vi "Insts_init.vi"(2 "Initialize sweep instruments ??":u64[](array[numeric]), 3 "sweep_list":string[](array[string])=["0:0"], 4 "Initialize readout instruments??":u64[](array[numeric]), 5 "Inst_array":T2(array[cluster])) -> (0 "Sweep inst parameters":T1(array[cluster]), 1 "Readout inst parameters":T1(array[cluster]))   [LabVIEW 2013]
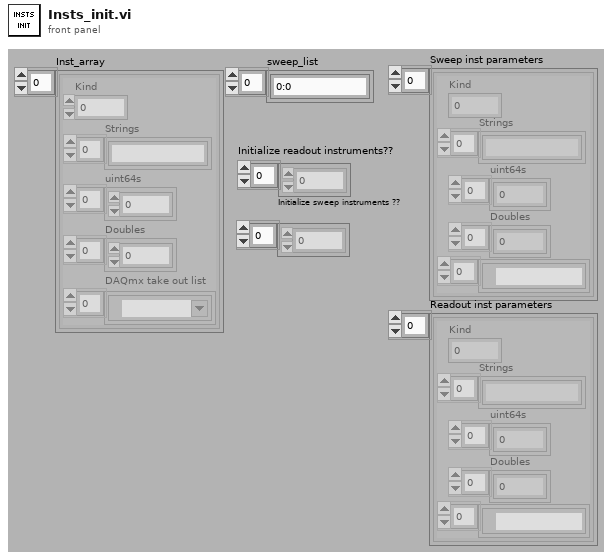
[diagram p1: front panel]
types:
  T1 = cluster{"Kind":u16, "Strings":string[], "uint64s":u64[], "Doubles":dbl[], refnum<k21>[]}[]
  T2 = cluster{"Kind":u16, "Strings":string[], "uint64s":u64[], "Doubles":dbl[], "DAQmx take out list":refnum<k21>[]}[]
  T3 = cluster{"Kind":u16, "Strings":string[], "uint64s":u64[], "Doubles":dbl[], refnum<k21>[]}
  T4 = cluster{"Kind":u16, "Strings":string[], "uint64s":u64[], "Doubles":dbl[], "DAQmx take out list":refnum<k21>[]}
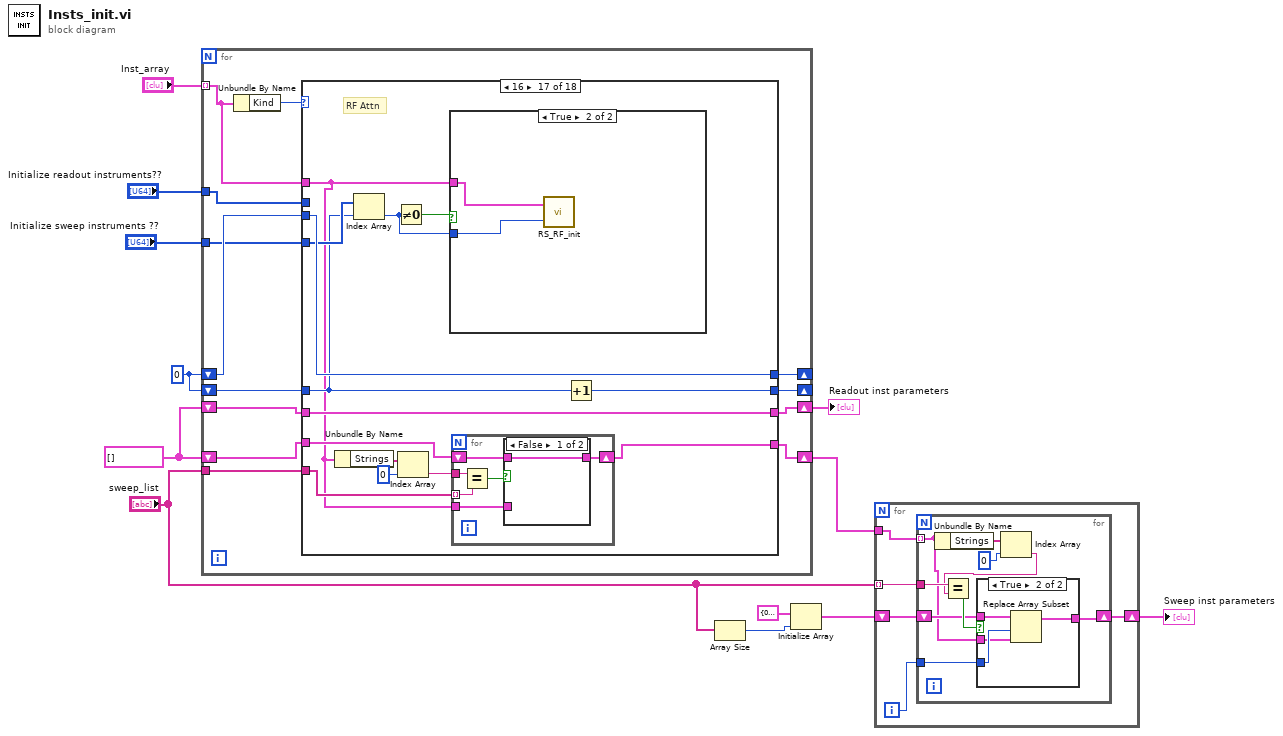
[diagram p0: block diagram]
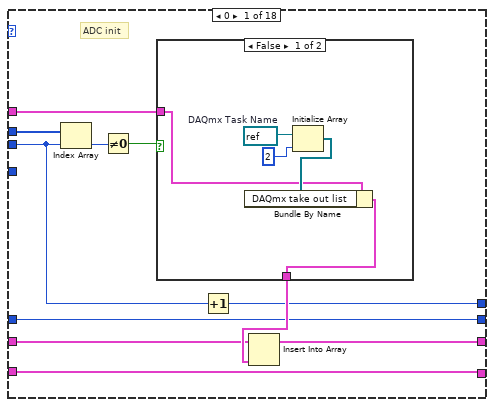
[diagram p3: hidden frame]
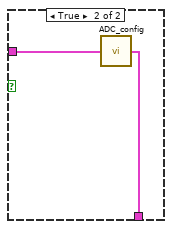
[diagram p4: hidden frame]
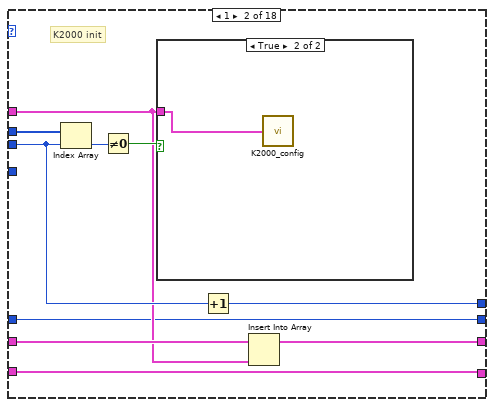
[diagram p5: hidden frame]
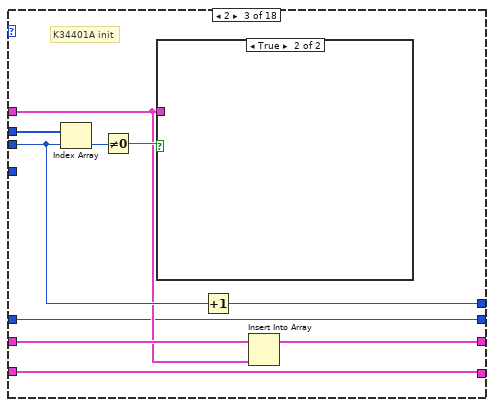
[diagram p7: hidden frame]
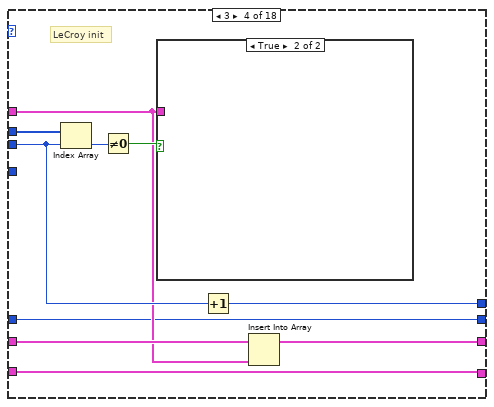
[diagram p9: hidden frame]
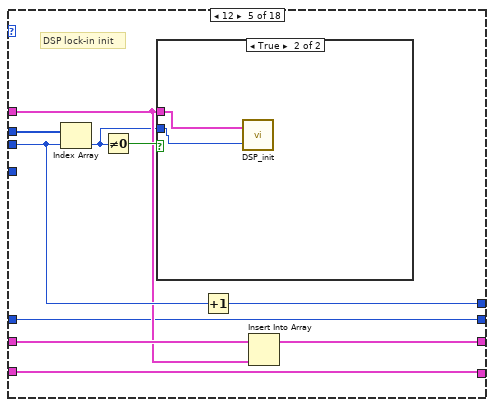
[diagram p11: hidden frame]
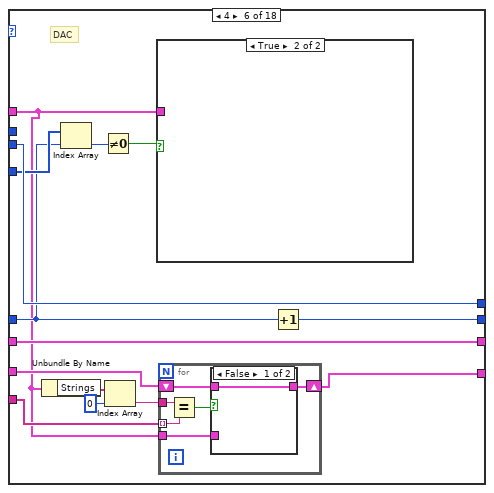
[diagram p13: hidden frame]
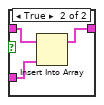
[diagram p14: hidden frame]
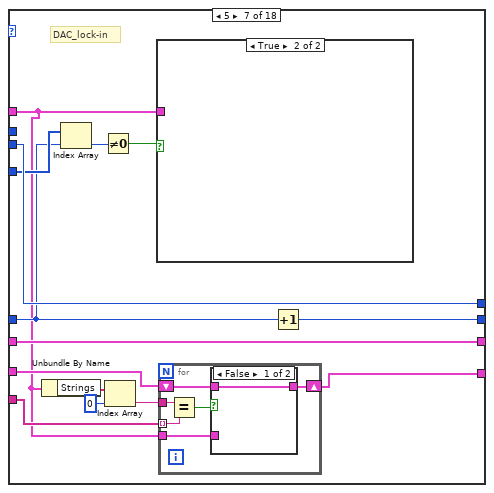
[diagram p16: hidden frame]
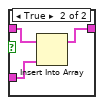
[diagram p17: hidden frame]
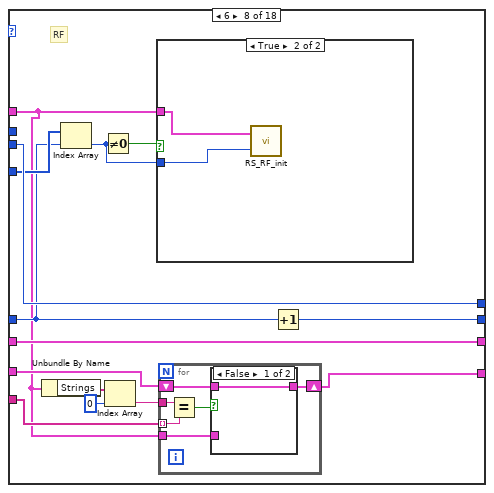
[diagram p19: hidden frame]
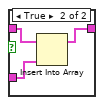
[diagram p20: hidden frame]
diagram:
  w9 = 0
  w8 = T1 [] ("Readout parameters")
  n1 = for {
    tunnel: "Inst_array" -> [w22] mode=indexing
    tunnel: "Initialize sweep instruments ??" -> [w19]
    tunnel: "Initialize readout instruments??" -> [w23]
    shift-right: [w13] -> w7
    shift-left: w8 -> [w16]
    shift-right: [w14] -> w2
    shift-left: w8 -> [w15]
    shift-right: [w21] -> _
    shift-left: w9 -> [w24]
    shift-right: [w18] -> _
    shift-left: w9 -> [w20]
    tunnel: "sweep_list" -> [w17]
    n2 = Unbundle By Name(w22) -> ("Kind"=w25:u16)
    n3 = case shown="16" w25 {
      tunnel: w24 -> [w31 w50 w61 w71 w82 w98 w122 w147 w173 w199 w223 w247 w271 w295 w319 w343 w369 w386]
      tunnel: w23 -> [w36 w53 w64 w74 w84 _ _ _ _ _ _ _ _ _ _ _ _ _]
      tunnel: w22 -> [w33 w46 w57 w67 w78 w87 w111 w136 w162 w188 w212 w236 w260 w284 w308 w332 w358 _]
      tunnel: [w30 w49 w60 w70 w81 w98 w122 w147 w173 w199 w223 w247 w271 w295 w319 w343 w369 w386] -> w21
      tunnel: w16 -> [w29 w48 w59 w69 w80 w95 w119 w144 w170 w196 w220 w244 w268 w292 w316 w340 w366 w385]
      tunnel: [w28 w47 w58 w68 w79 w95 w119 w144 w170 w196 w220 w244 w268 w292 w316 w340 w366 w385] -> w13
      tunnel: w20 -> [w27 w45 w56 w66 w77 w94 w118 w143 w169 w195 w219 w243 w267 w291 w315 w339 w365 w384]
      tunnel: w19 -> [_ _ _ _ _ w97 w121 w146 w172 w198 w222 w246 w270 w294 w318 w342 w368 _]
      tunnel: [w27 w45 w56 w66 w77 w96 w120 w145 w171 w197 w221 w245 w269 w293 w317 w341 w367 w384] -> w18
      tunnel: w15 -> [w26 w44 w55 w65 w76 w89 w113 w138 w164 w190 w214 w238 w262 w286 w310 w334 w360 w383]
      tunnel: [w26 w44 w55 w65 w76 w88 w112 w137 w163 w189 w213 w237 w261 w285 w309 w333 w359 w383] -> w14
      tunnel: w17 -> [_ _ _ _ _ w90 w114 w139 w165 w191 w215 w239 w263 w287 w311 w335 w361 _]
      frame 0 {
        # "ADC init"
        n4 = Index Array(array=w36, index=w31) -> (element=w35:u64)
        n5 = Not Equal To 0?(x=w35) -> (x != 0?=w34:bool)
        n6 = case shown="False" w34 {
          tunnel: w33 -> [w38 w43]
          tunnel: [w37 w42] -> w32
          frame False {
            w41 = refnum<k21> refnum  # DAQmx Task Name
            n7 = Initialize Array(w41, 2) -> (w39:refnum<k21>[])
            n8 = Bundle By Name(cluster=w38, "DAQmx take out list"=w39) -> (w37:T4)
          }
          frame True {
            n9 = call "ADC_config.vi"("Inst_parameter"=w43) -> ("Inst_parameter out"=w42:T4)
          }
        }
        n10 = Increment(x=w31) -> (x+1=w30:i32)
        n11 = Insert Into Array(array=w29, new element=w32) -> (w28:T1)  [unwired: 1 in]
      }
      frame 1 {
        # "K2000 init"
        n12 = Index Array(array=w53, index=w50) -> (element=w52:u64)
        n13 = Not Equal To 0?(x=w52) -> (x != 0?=w51:bool)
        n14 = case shown="True" w51 {
          tunnel: w46 -> [_ w54]
          frame False {
          }
          frame True {
            n15 = call "K2000_config.vi"("Readout_inst_parameters"=w54) -> ()  [unwired: 1 out]
          }
        }
        n16 = Increment(x=w50) -> (x+1=w49:i32)
        n17 = Insert Into Array(array=w48, new element=w46) -> (w47:T1)  [unwired: 1 in]
      }
      frame 2 {
        # "K34401A init"
        n18 = Index Array(array=w64, index=w61) -> (element=w63:u64)
        n19 = Not Equal To 0?(x=w63) -> (x != 0?=w62:bool)
        n20 = case shown="True" w62 {
          tunnel: w57 -> [_ _]
          frame False {
          }
          frame True {
          }
        }
        n21 = Increment(x=w61) -> (x+1=w60:i32)
        n22 = Insert Into Array(array=w59, new element=w57) -> (w58:T1)  [unwired: 1 in]
      }
      frame 3 {
        # "LeCroy init"
        n23 = Index Array(array=w74, index=w71) -> (element=w73:u64)
        n24 = Not Equal To 0?(x=w73) -> (x != 0?=w72:bool)
        n25 = case shown="True" w72 {
          tunnel: w67 -> [_ _]
          frame False {
          }
          frame True {
          }
        }
        n26 = Increment(x=w71) -> (x+1=w70:i32)
        n27 = Insert Into Array(array=w69, new element=w67) -> (w68:T1)  [unwired: 1 in]
      }
      frame 12 {
        # "DSP lock-in init"
        n28 = Index Array(array=w84, index=w82) -> (element=w75:u64)
        n29 = Not Equal To 0?(x=w75) -> (x != 0?=w83:bool)
        n30 = case shown="True" w83 {
          tunnel: w78 -> [_ w86]
          tunnel: w75 -> [_ w85]
          frame False {
          }
          frame True {
            n31 = call "DSP_init.vi"("Initialize Instrument"=w85, "Inst_param"=w86) -> ()  [unwired: 1 in]
          }
        }
        n32 = Increment(x=w82) -> (x+1=w81:i32)
        n33 = Insert Into Array(array=w80, new element=w78) -> (w79:T1)  [unwired: 1 in]
      }
      frame 4 {
        # "DAC"
        n34 = Unbundle By Name(w87) -> ("Strings"=w93:string[])
        n35 = Index Array(array=w97, index=w94) -> (element=w100:u64)
        n36 = Not Equal To 0?(x=w100) -> (x != 0?=w99:bool)
        n37 = Index Array(array=w93, index=0) -> (element=w91:string)
        n38 = case shown="True" w99 {
          tunnel: w87 -> [_ _]
          frame False {
          }
          frame True {
          }
        }
        n39 = for {
          tunnel: w91 -> [w106]
          tunnel: w90 -> [w105] mode=indexing
          shift-right: [w101] -> w88
          shift-left: w89 -> [w102]
          tunnel: w87 -> [w103]
          n40 = Equal?(x=w106, y=w105) -> (x = y?=w104:bool)
          n41 = case shown="False" w104 {
            tunnel: w103 -> [_ w110]
            tunnel: w102 -> [w107 w109]
            tunnel: [w107 w108] -> w101
            frame False {
            }
            frame True {
              n42 = Insert Into Array(array=w109, new element=w110) -> (w108:T1)  [unwired: 1 in]
            }
          }
        }
        n43 = Increment(x=w94) -> (x+1=w96:i32)
      }
      frame 5 {
        # "DAC_lock-in"
        n44 = Unbundle By Name(w111) -> ("Strings"=w117:string[])
        n45 = Index Array(array=w121, index=w118) -> (element=w124:u64)
        n46 = Not Equal To 0?(x=w124) -> (x != 0?=w123:bool)
        n47 = Index Array(array=w117, index=0) -> (element=w115:string)
        n48 = case shown="True" w123 {
          tunnel: w111 -> [_ _]
          frame False {
          }
          frame True {
          }
        }
        n49 = for {
          tunnel: w115 -> [w130]
          tunnel: w114 -> [w129] mode=indexing
          shift-right: [w125] -> w112
          shift-left: w113 -> [w126]
          tunnel: w111 -> [w127]
          n50 = Equal?(x=w130, y=w129) -> (x = y?=w128:bool)
          n51 = case shown="False" w128 {
            tunnel: w127 -> [_ w134]
            tunnel: w126 -> [w131 w133]
            tunnel: [w131 w132] -> w125
            frame False {
            }
            frame True {
              n52 = Insert Into Array(array=w133, new element=w134) -> (w132:T1)  [unwired: 1 in]
            }
          }
        }
        n53 = Increment(x=w118) -> (x+1=w120:i32)
      }
      frame 6 {
        # "RF"
        n54 = Unbundle By Name(w136) -> ("Strings"=w142:string[])
        n55 = Index Array(array=w146, index=w143) -> (element=w135:u64)
        n56 = Not Equal To 0?(x=w135) -> (x != 0?=w148:bool)
        n57 = Index Array(array=w142, index=0) -> (element=w140:string)
        n58 = case shown="True" w148 {
          tunnel: w136 -> [_ w160]
          tunnel: w135 -> [_ w159]
          frame False {
          }
          frame True {
            n59 = call "RS_RF_init.vi"("Initialize Instrument"=w159, "Inst_param"=w160) -> ()  [unwired: 1 in]
          }
        }
        n60 = for {
          tunnel: w140 -> [w154]
          tunnel: w139 -> [w153] mode=indexing
          shift-right: [w149] -> w137
          shift-left: w138 -> [w150]
          tunnel: w136 -> [w151]
          n61 = Equal?(x=w154, y=w153) -> (x = y?=w152:bool)
          n62 = case shown="False" w152 {
            tunnel: w151 -> [_ w158]
            tunnel: w150 -> [w155 w157]
            tunnel: [w155 w156] -> w149
            frame False {
            }
            frame True {
              n63 = Insert Into Array(array=w157, new element=w158) -> (w156:T1)  [unwired: 1 in]
            }
          }
        }
        n64 = Increment(x=w143) -> (x+1=w145:i32)
      }
      frame 7 {
        # "AWG"
        n65 = Unbundle By Name(w162) -> ("Strings"=w168:string[])
        n66 = Index Array(array=w172, index=w169) -> (element=w161:u64)
        n67 = Not Equal To 0?(x=w161) -> (x != 0?=w174:bool)
        n68 = Index Array(array=w168, index=0) -> (element=w166:string)
        n69 = case shown="True" w174 {
          tunnel: w162 -> [_ w186]
          tunnel: w161 -> [_ w185]
          frame False {
          }
          frame True {
            n70 = call "AWG_init.vi"("Initialize?"=w185, "Inst_param"=w186) -> ()  [unwired: 1 out]
          }
        }
        n71 = for {
          tunnel: w166 -> [w180]
          tunnel: w165 -> [w179] mode=indexing
          shift-right: [w175] -> w163
          shift-left: w164 -> [w176]
          tunnel: w162 -> [w177]
          n72 = Equal?(x=w180, y=w179) -> (x = y?=w178:bool)
          n73 = case shown="False" w178 {
            tunnel: w177 -> [_ w184]
            tunnel: w176 -> [w181 w183]
            tunnel: [w181 w182] -> w175
            frame False {
            }
            frame True {
              n74 = Insert Into Array(array=w183, new element=w184) -> (w182:T1)  [unwired: 1 in]
            }
          }
        }
        n75 = Increment(x=w169) -> (x+1=w171:i32)
      }
      frame 8 {
        # "B-field"
        n76 = Unbundle By Name(w188) -> ("Strings"=w194:string[])
        n77 = Index Array(array=w198, index=w195) -> (element=w187:u64)
        n78 = Not Equal To 0?(x=w187) -> (x != 0?=w200:bool)
        n79 = Index Array(array=w194, index=0) -> (element=w192:string)
        n80 = case shown="True" w200 {
          tunnel: w188 -> [_ _]
          tunnel: w187 -> [_ _]
          frame False {
          }
          frame True {
          }
        }
        n81 = for {
          tunnel: w192 -> [w206]
          tunnel: w191 -> [w205] mode=indexing
          shift-right: [w201] -> w189
          shift-left: w190 -> [w202]
          tunnel: w188 -> [w203]
          n82 = Equal?(x=w206, y=w205) -> (x = y?=w204:bool)
          n83 = case shown="False" w204 {
            tunnel: w203 -> [_ w210]
            tunnel: w202 -> [w207 w209]
            tunnel: [w207 w208] -> w201
            frame False {
            }
            frame True {
              n84 = Insert Into Array(array=w209, new element=w210) -> (w208:T1)  [unwired: 1 in]
            }
          }
        }
        n85 = Increment(x=w195) -> (x+1=w197:i32)
      }
      frame 9 {
        # "Fast sequence"
        n86 = Unbundle By Name(w212) -> ("Strings"=w218:string[])
        n87 = Index Array(array=w222, index=w219) -> (element=w211:u64)
        n88 = Not Equal To 0?(x=w211) -> (x != 0?=w224:bool)
        n89 = Index Array(array=w218, index=0) -> (element=w216:string)
        n90 = case shown="True" w224 {
          tunnel: w212 -> [_ _]
          tunnel: w211 -> [_ _]
          frame False {
          }
          frame True {
          }
        }
        n91 = for {
          tunnel: w216 -> [w230]
          tunnel: w215 -> [w229] mode=indexing
          shift-right: [w225] -> w213
          shift-left: w214 -> [w226]
          tunnel: w212 -> [w227]
          n92 = Equal?(x=w230, y=w229) -> (x = y?=w228:bool)
          n93 = case shown="False" w228 {
            tunnel: w227 -> [_ w234]
            tunnel: w226 -> [w231 w233]
            tunnel: [w231 w232] -> w225
            frame False {
            }
            frame True {
              n94 = Insert Into Array(array=w233, new element=w234) -> (w232:T1)  [unwired: 1 in]
            }
          }
        }
        n95 = Increment(x=w219) -> (x+1=w221:i32)
      }
      frame 10 {
        # "Fast sequence slot"
        n96 = Unbundle By Name(w236) -> ("Strings"=w242:string[])
        n97 = Index Array(array=w246, index=w243) -> (element=w235:u64)
        n98 = Not Equal To 0?(x=w235) -> (x != 0?=w248:bool)
        n99 = Index Array(array=w242, index=0) -> (element=w240:string)
        n100 = case shown="True" w248 {
          tunnel: w236 -> [_ _]
          tunnel: w235 -> [_ _]
          frame False {
          }
          frame True {
          }
        }
        n101 = for {
          tunnel: w240 -> [w254]
          tunnel: w239 -> [w253] mode=indexing
          shift-right: [w249] -> w237
          shift-left: w238 -> [w250]
          tunnel: w236 -> [w251]
          n102 = Equal?(x=w254, y=w253) -> (x = y?=w252:bool)
          n103 = case shown="False" w252 {
            tunnel: w251 -> [_ w258]
            tunnel: w250 -> [w255 w257]
            tunnel: [w255 w256] -> w249
            frame False {
            }
            frame True {
              n104 = Insert Into Array(array=w257, new element=w258) -> (w256:T1)  [unwired: 1 in]
            }
          }
        }
        n105 = Increment(x=w243) -> (x+1=w245:i32)
      }
      frame 11 {
        # "Command line"
        n106 = Unbundle By Name(w260) -> ("Strings"=w266:string[])
        n107 = Index Array(array=w270, index=w267) -> (element=w259:u64)
        n108 = Not Equal To 0?(x=w259) -> (x != 0?=w272:bool)
        n109 = Index Array(array=w266, index=0) -> (element=w264:string)
        n110 = case shown="True" w272 {
          tunnel: w260 -> [_ _]
          tunnel: w259 -> [_ _]
          frame False {
          }
          frame True {
          }
        }
        n111 = for {
          tunnel: w264 -> [w278]
          tunnel: w263 -> [w277] mode=indexing
          shift-right: [w273] -> w261
          shift-left: w262 -> [w274]
          tunnel: w260 -> [w275]
          n112 = Equal?(x=w278, y=w277) -> (x = y?=w276:bool)
          n113 = case shown="False" w276 {
            tunnel: w275 -> [_ w282]
            tunnel: w274 -> [w279 w281]
            tunnel: [w279 w280] -> w273
            frame False {
            }
            frame True {
              n114 = Insert Into Array(array=w281, new element=w282) -> (w280:T1)  [unwired: 1 in]
            }
          }
        }
        n115 = Increment(x=w267) -> (x+1=w269:i32)
      }
      frame 13 {
        # "DSP lock-in sweep"
        n116 = Unbundle By Name(w284) -> ("Strings"=w290:string[])
        n117 = Index Array(array=w294, index=w291) -> (element=w283:u64)
        n118 = Not Equal To 0?(x=w283) -> (x != 0?=w296:bool)
        n119 = Index Array(array=w290, index=0) -> (element=w288:string)
        n120 = case shown="True" w296 {
          tunnel: w284 -> [_ _]
          tunnel: w283 -> [_ _]
          frame False {
          }
          frame True {
          }
        }
        n121 = for {
          tunnel: w288 -> [w302]
          tunnel: w287 -> [w301] mode=indexing
          shift-right: [w297] -> w285
          shift-left: w286 -> [w298]
          tunnel: w284 -> [w299]
          n122 = Equal?(x=w302, y=w301) -> (x = y?=w300:bool)
          n123 = case shown="False" w300 {
            tunnel: w299 -> [_ w306]
            tunnel: w298 -> [w303 w305]
            tunnel: [w303 w304] -> w297
            frame False {
            }
            frame True {
              n124 = Insert Into Array(array=w305, new element=w306) -> (w304:T1)  [unwired: 1 in]
            }
          }
        }
        n125 = Increment(x=w291) -> (x+1=w293:i32)
      }
      frame 14 {
        # "ms to wait"
        n126 = Unbundle By Name(w308) -> ("Strings"=w314:string[])
        n127 = Index Array(array=w318, index=w315) -> (element=w307:u64)
        n128 = Not Equal To 0?(x=w307) -> (x != 0?=w320:bool)
        n129 = Index Array(array=w314, index=0) -> (element=w312:string)
        n130 = case shown="True" w320 {
          tunnel: w308 -> [_ _]
          tunnel: w307 -> [_ _]
          frame False {
          }
          frame True {
          }
        }
        n131 = for {
          tunnel: w312 -> [w326]
          tunnel: w311 -> [w325] mode=indexing
          shift-right: [w321] -> w309
          shift-left: w310 -> [w322]
          tunnel: w308 -> [w323]
          n132 = Equal?(x=w326, y=w325) -> (x = y?=w324:bool)
          n133 = case shown="False" w324 {
            tunnel: w323 -> [_ w330]
            tunnel: w322 -> [w327 w329]
            tunnel: [w327 w328] -> w321
            frame False {
            }
            frame True {
              n134 = Insert Into Array(array=w329, new element=w330) -> (w328:T1)  [unwired: 1 in]
            }
          }
        }
        n135 = Increment(x=w315) -> (x+1=w317:i32)
      }
      frame 15 {
        # "ATM delay line"
        n136 = Unbundle By Name(w332) -> ("Strings"=w338:string[])
        n137 = Index Array(array=w342, index=w339) -> (element=w331:u64)
        n138 = Not Equal To 0?(x=w331) -> (x != 0?=w344:bool)
        n139 = Index Array(array=w338, index=0) -> (element=w336:string)
        n140 = case shown="True" w344 {
          tunnel: w332 -> [_ w356]
          tunnel: w331 -> [_ w355]
          frame False {
          }
          frame True {
            n141 = call "DelayLineInit.vi"("Inst bool"=w355, "Inst_param"=w356) -> ()  [unwired: 1 in]
          }
        }
        n142 = for {
          tunnel: w336 -> [w350]
          tunnel: w335 -> [w349] mode=indexing
          shift-right: [w345] -> w333
          shift-left: w334 -> [w346]
          tunnel: w332 -> [w347]
          n143 = Equal?(x=w350, y=w349) -> (x = y?=w348:bool)
          n144 = case shown="False" w348 {
            tunnel: w347 -> [_ w354]
            tunnel: w346 -> [w351 w353]
            tunnel: [w351 w352] -> w345
            frame False {
            }
            frame True {
              n145 = Insert Into Array(array=w353, new element=w354) -> (w352:T1)  [unwired: 1 in]
            }
          }
        }
        n146 = Increment(x=w339) -> (x+1=w341:i32)
      }
      frame 16 {
        # "RF Attn"
        n147 = Unbundle By Name(w358) -> ("Strings"=w364:string[])
        n148 = Index Array(array=w368, index=w365) -> (element=w357:u64)
        n149 = Not Equal To 0?(x=w357) -> (x != 0?=w370:bool)
        n150 = Index Array(array=w364, index=0) -> (element=w362:string)
        n151 = case shown="True" w370 {
          tunnel: w358 -> [_ w382]
          tunnel: w357 -> [_ w381]
          frame False {
          }
          frame True {
            n152 = call "RS_RF_init.vi"("Initialize Instrument"=w381, "Inst_param"=w382) -> ()  [unwired: 1 in]
          }
        }
        n153 = for {
          tunnel: w362 -> [w376]
          tunnel: w361 -> [w375] mode=indexing
          shift-right: [w371] -> w359
          shift-left: w360 -> [w372]
          tunnel: w358 -> [w373]
          n154 = Equal?(x=w376, y=w375) -> (x = y?=w374:bool)
          n155 = case shown="False" w374 {
            tunnel: w373 -> [_ w380]
            tunnel: w372 -> [w377 w379]
            tunnel: [w377 w378] -> w371
            frame False {
            }
            frame True {
              n156 = Insert Into Array(array=w379, new element=w380) -> (w378:T1)  [unwired: 1 in]
            }
          }
        }
        n157 = Increment(x=w365) -> (x+1=w367:i32)
      }
      frame 100, Default {
        # "Else"
      }
    }
  }
  "Readout inst parameters" <- w7
  n158 = Array Size(array="sweep_list") -> (size(s)=w4:i32)
  n159 = Initialize Array(T3 {"Kind"=0, "Strings"=[], "uint64s"=[], "Doubles"=[], []}, w4) -> (w3:T1)
  n160 = for {
    tunnel: "sweep_list" -> [w389] mode=indexing
    tunnel: w2 -> [w388]
    shift-right: [w387] -> w1
    shift-left: w3 -> [w391]
    i -> [w390]
    n161 = for {
      shift-right: [w394] -> w387
      shift-left: w391 -> [w395]
      tunnel: w390 -> [w393]
      tunnel: w389 -> [w398]
      tunnel: w388 -> [w392] mode=indexing
      n162 = Unbundle By Name(w392) -> ("Strings"=w400:string[])
      n163 = Index Array(array=w400, index=0) -> (element=w397:string)
      n164 = Equal?(x=w398, y=w397) -> (x = y?=w396:bool)
      n165 = case shown="True" w396 {
        tunnel: w395 -> [w401 w405]
        tunnel: [w401 w404] -> w394
        tunnel: w393 -> [_ w403]
        tunnel: w392 -> [_ w402]
        frame False {
        }
        frame True {
          n166 = Replace Array Subset(array=w405, new element=w402, index=w403) -> (w404:T1)
        }
      }
    }
  }
  "Sweep inst parameters" <- w1
